vi "Count_Events.vi"(8 "error in (no error)":errorcluster, 10 "Small?":bool, 11 "Constraints":T1 {"Estimate Quality" scale=0.0..5.0; "Lower Mass Limit (kg)" min=-1.0 max=1.0 step=1e-20; "Upper Mass Limit (kg)" min=-1.0 max=1.0 step=1e-20; "Lower Velocity Limit (km/s)" min=-1.0 max=299792000.0; "Upper Velocity Limit (km/s)" min=-1.0 max=299792000.0}) -> (0 "error out":errorcluster, 3 "Number of Events":u64)   [LabVIEW 2013]
uses:
  User Interface/Controls/Constraints.ctl
  <vilib>/addons/database/_DB Variant To Data/Database Variant To Data.xnode
panel:
  out "Count Events Syntax":string
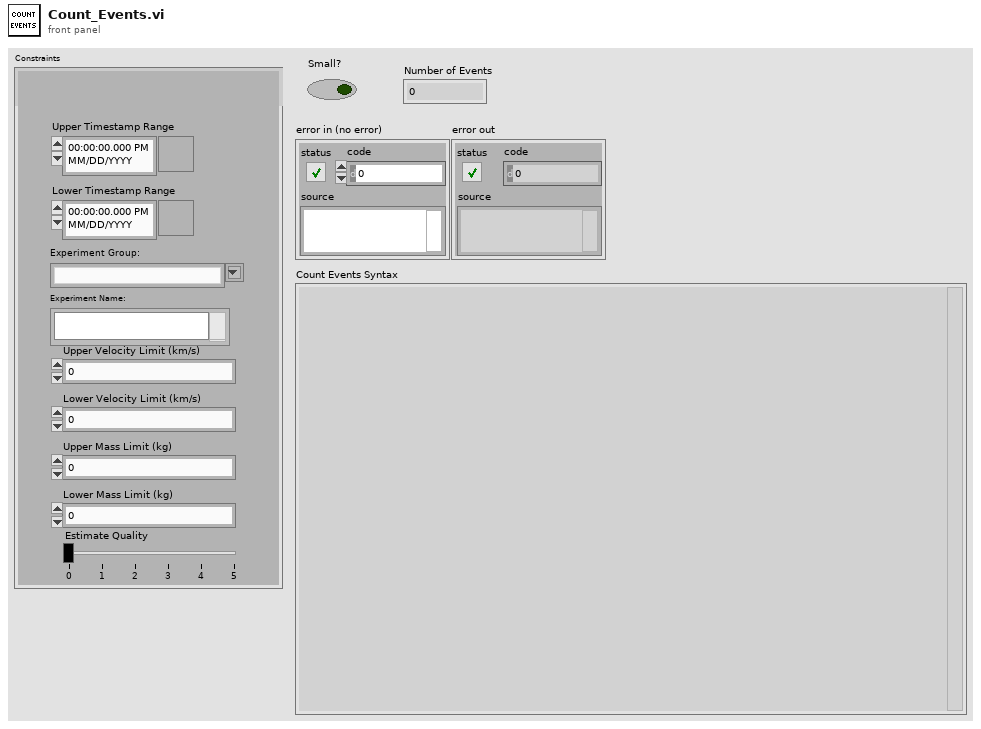
[diagram p1: front panel]
types:
  T1 = typedef "Constraints.ctl" = cluster{"Upper Timestamp Range":timestamp, "Lower Timestamp Range":timestamp, "Experiment Group:":string, "Experiment Name:":i32[], "Upper Velocity Limit (km/s)":dbl, "Lower Velocity Limit (km/s)":dbl, "Upper Mass Limit (kg)":dbl, "Lower Mass Limit (kg)":dbl, "name array":string[], "Estimate Quality":cluster{dbl, dbl}}
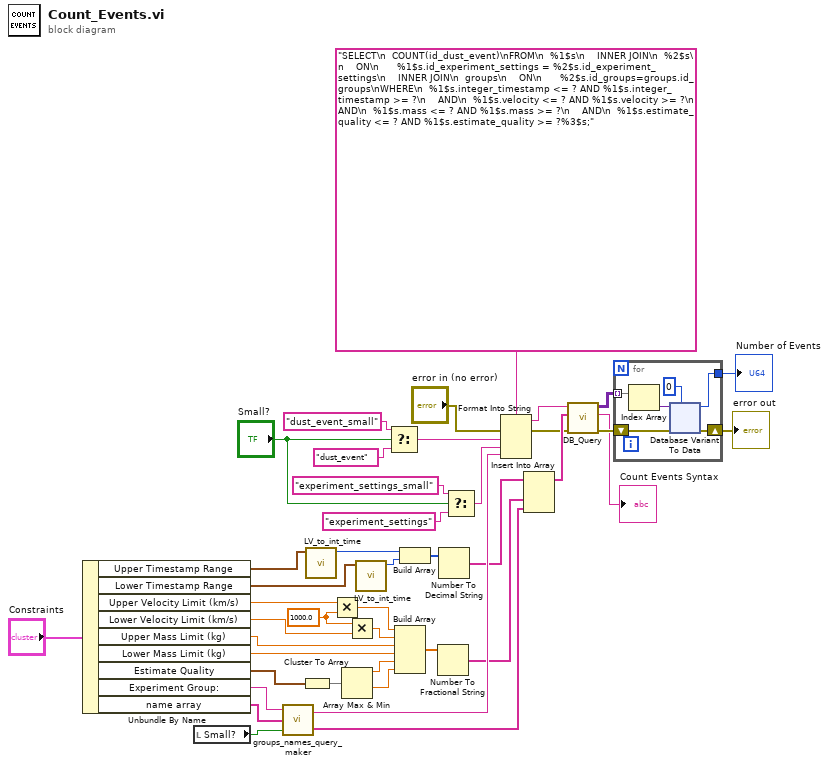
[diagram p0: block diagram]
diagram:
  w41 = 1000.0 ("y")
  n1 = Unbundle By Name("Constraints") -> ("Upper Timestamp Range"=w24:timestamp, "Lower Timestamp Range"=w23:timestamp, "Upper Velocity Limit (km/s)"=w26:dbl, "Lower Velocity Limit (km/s)"=w25:dbl, "Upper Mass Limit (kg)"=w12:dbl, "Lower Mass Limit (kg)"=w13:dbl, "Estimate Quality"=w28:cluster{dbl, dbl}, "Experiment Group:"=w32:string, "name array"=w27:string[])
  n2 = local read "Small?"() -> (w33:bool)
  n3 = call "groups_names_query_maker.vi"("Small?"=w33, "Name Array"=w27, "Group  Name"=w32) -> ("Parameters"=w1:string[], "Group and Names Query"=w22:string)
  n4 = Cluster To Array(cluster=w28) -> (array=w42:dbl[])
  n5 = call "LV_to_int_time.vi"("Time Stamp"=w24) -> ("Integer Time"=w8:i64)  [unwired: 8 in, 1 out]
  n6 = Multiply(x=w26, y=w41) -> (x*y=w10:dbl)
  n7 = Array Max & Min(array=w42) -> (max value=w15:dbl, min value=w14:dbl)  [unwired: 2 out]
  n8 = Multiply(x=w41, y=w25) -> (x*y=w11:dbl)
  n9 = call "LV_to_int_time.vi"("Time Stamp"=w23) -> ("Integer Time"=w9:i64)  [unwired: 8 in, 1 out]
  n10 = Select(t="dust_event_small" ("string"), s="Small?", f="dust_event" ("string")) -> (s? t:f=w30:string)
  n11 = Build Array(w10, w11, w12, w13, w15, w14) -> (w7:dbl[])
  n12 = Build Array(w8, w9) -> (w6:i64[])
  n13 = Number To Fractional String(number=w7) -> (F-format string=w2:string[])  [unwired: 3 in]
  n14 = Number To Decimal String(number=w6) -> (decimal integer string=w3:string[])  [unwired: 1 in]
  n15 = Select(t="experiment_settings_small" ("string"), s="Small?", f="experiment_settings" ("string")) -> (s? t:f=w17:string)
  n16 = Format Into String(format string="SELECT\n  COUNT(id_dust_event)\nFROM\n  %1$s\n    INNER JOIN\n  %2$s\n    ON\n      %1$s.id_experiment_settings = %2$s.id_experiment_settings\n    INNER JOIN\n  groups\n    ON\n      %2$s.id_groups=groups.id_groups\nWHERE\n  %1$s.integer_timestamp <= ? AND %1$s.integer_timestamp >= ?\n    AND\n  %1$s.velocity <= ? AND %1$s.velocity >= ?\n    AND\n  %1$s.mass <= ? AND %1$s.mass >= ?\n    AND\n  %1$s.estimate_quality <= ? AND %1$s.estimate_quality >= ?%3$s;" ("string"), error in="error in (no error)", w30, w17, w22) -> (resulting string=w29:string, error out=w4:errorcluster)  [unwired: 1 in]
  n17 = Insert Into Array(array=w3, new element #1=w2, new element #2=w1) -> (w16:string[])  [unwired: 1 in]
  n18 = call "DB_Query.vi"("error in (no error)"=w4, "Parameters"=w16, "Parameterized Query"=w29) -> ("error out"=w36:errorcluster, "Query in Standard Format"=→"Count Events Syntax":string, "Results"=w35:variant[][])  [unwired: 6 in]
  n19 = for {
    tunnel: [w47] -> w38
    tunnel: w35 -> [w43] mode=indexing
    shift-right: [w48] -> w39
    shift-left: w36 -> [w45]
    n20 = Index Array(array=w43) -> (element=w44:variant)  [unwired: 1 in]
    n21 = xnode "Database Variant To Data"("database variant"=w44, "error in (no error)"=w45, "type"=u64 0 ("Number of Events")) -> ("data"=w47:u64, "error out"=w48:errorcluster)
  }
  "error out" <- w39
  "Number of Events" <- w38
